vi "Stereo - Grid Parameters Dialog.vi"() -> (0 "Cancel Indicator":bool, 2 "Grid Size out":cluster{"X":i32, "Y":i32}, 3 "Grid Descriptor out":cluster{"X Step":sgl, "Y Step":sgl, "Unit":T1}={"X Step"=1.0, "Y Step"=1.0, "Unit"=enum."Inch"})   [LabVIEW 2014]
doc: "Dialog to let the user specify the grid parameters."
panel:
  in  "OK":bool
  in  "Grid Descriptor in":cluster{"X Step":sgl, "Y Step":sgl, "Unit":u16}={"X Step"=1.0, "Y Step"=1.0, "Unit"=8} caption="Grid Descriptor" {"Unit" items=["Undefined", "Angström", "Micrometer", "Millimeter", "Centimeter", "Meter", "Kilometer", "Microinch", "Inch", "Feet", "Nautical miles", "Standard miles", "Steps"]; "Y Step" min=9 format="%#.2g"; "X Step" min=0 format="%#.2g"}
  in  "Cancel":bool
  in  "Grid Size in":cluster{"X":i32, "Y":i32}={"X"=29, "Y"=19} caption="Grid Size" {"Y" min=9; "X" min=9}
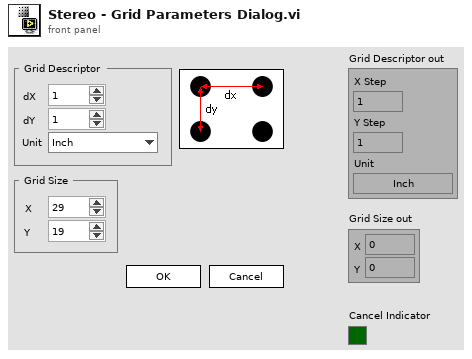
[diagram p1: front panel]
types:
  T1 = typedef "Image Unit" = enum32{"Undefined", "Angström", "Micrometer", "Millimeter", "Centimeter", "Meter", "Kilometer", "Microinch", "Inch", "Feet", "Nautical miles", "Standard miles", "Steps"}
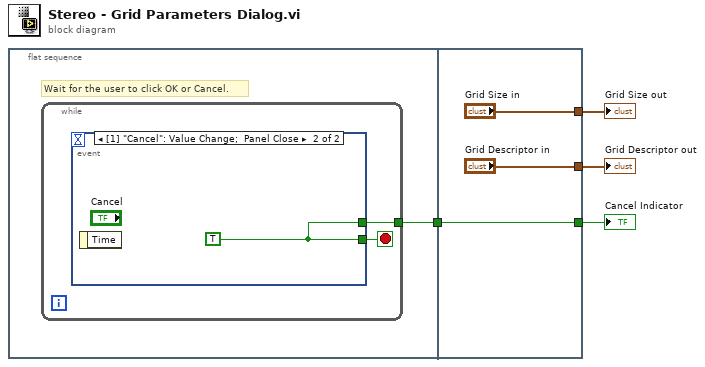
[diagram p0: block diagram]
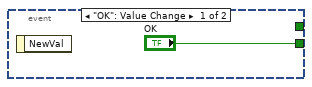
[diagram p2: hidden frame]
diagram:
  n1 = flat-sequence {
    tunnel: [w5] -> w3
    tunnel: [w12] -> w4
    tunnel: w3 -> [w12]
    tunnel: ["Grid Size in"] -> w2
    tunnel: ["Grid Descriptor in"] -> w1
    frame #0 {
      # "Wait for the user to click OK or Cancel."
      n2 = while {
        tunnel: [w6] -> w5
        stop <- w7 stop-if-true
        n3 = event shown="[1] \"Cancel\": Value Change;  Panel Close" {
          selector: _ -> [_ _]
          dyn-events: _ -> [_ _]
          timeout: _ -> [_ _]
          tunnel: ["OK" w9] -> w7
          tunnel: [_ w9] -> w6
          event "OK": Value Change {
            n4 = event-data() -> ()  [unwired: 2 out]
          }
          event "Cancel": Value Change; Panel Close {
            w9 = TRUE ("NewVal")
            n5 = event-data() -> ()  [unwired: 2 out]
          }
        }
      }
    }
    frame #1 {
    }
  }
  "Grid Descriptor out" <- w1
  "Grid Size out" <- w2
  "Cancel Indicator" <- w4
